vi "TempLog.vi"   [LabVIEW 2014]
uses:
  <vilib>/Utility/file.llb/Write To Spreadsheet File (DBL).vi
types:
  T1 = cluster{"refnum name":string, "refnum name":string, "refnum name":string, "refnum name":string}
  T2 = typedef "WPI_AnalogChannelDevRef.ctl" = cluster{"DevStatus":errorcluster, "Controller":T3, "Analog Channel":T4}
  T3 = typedef "FPGA_TypedefAnalogModule.ctl" = enum16{"Controller 1"}
  T4 = typedef "FPGA_AIChannel.ctl" = enum8{"AI 0", "AI 1", "AI 2", "AI 3", "AI MXP 0", "AI MXP 1", "AI MXP 2", "AI MXP 3", "Invalid"}
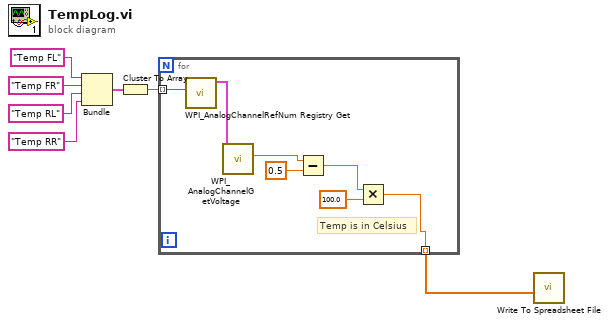
[diagram p0: block diagram]
diagram:
  n1 = Bundle("refnum name"="Temp FL", "refnum name"="Temp FR", "refnum name"="Temp RL", "refnum name"="Temp RR") -> (w3:T1)  [unwired: 1 in]
  n2 = Cluster To Array(cluster=w3) -> (array=w2:string[])
  n3 = for {
    tunnel: w2 -> [w14] mode=indexing
    tunnel: [w11] -> w1 mode=indexing
    # "Temp is in Celsius"
    n4 = call <vilib>:"WPI_AnalogChannelRefNum Registry Get.vi"("refnum name"=w14) -> ("AIDeviceRef"=w13:T2)  [unwired: 9 in, 1 out]
    n5 = call <vilib>:"WPI_AnalogChannelGetVoltage.vi"("AIDeviceRef"=w13) -> ("Voltage"=w8:dbl)  [unwired: 8 in, 2 out]
    n6 = Subtract(x=w8, y=0.5) -> (x-y=w12:dbl)
    n7 = Multiply(x=w12, y=100.0) -> (x*y=w11:dbl)
  }
  n8 = call-poly <vilib>:"Write To Spreadsheet File.vi"("1D data"=w1) -> ()  [unwired: 7 in, 1 out]
